vi "Asylum_Driver_LithographyObjectPoints.vi"(6 "Interpolation":dbl format="%#_13g", 7 "Writing Setpoint":dbl=0.1 format="%#_13g", 8 "error in (no error)":errorcluster, 9 "Offsets":cluster{"X":dbl, "Y":dbl}, 10 "Pattern Data":T2={"Name"="", "Litho"=[], "Set Resistance"=enum."1G ohm"}, 11 "Application":refnum<k7>) -> (0 "error out":errorcluster, 3 "Application":refnum<k7>)   [LabVIEW 2020]
uses:
  Asylum_Driver_XYMetersToVoltageArray.vi
  <userlib>/LevyLab/Relay Box/Type_defs/Resistor--enum.ctl
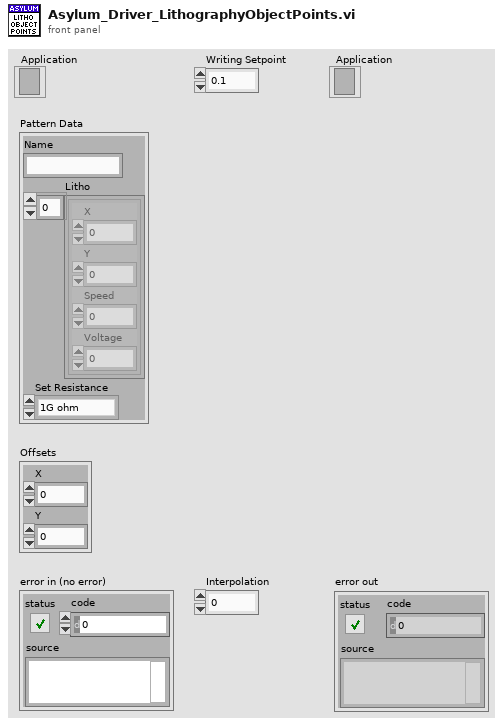
[diagram p1: front panel]
types:
  T1 = typedef "Resistor--enum.ctl" = enum16{"open", "discharge tip", "0 ohms", "100k ohm", "10M ohm", "1G ohm"}
  T2 = cluster{"Name":string, "Litho":cluster{"X":dbl, "Y":dbl, "Speed":dbl, "Voltage":dbl}[], "Set Resistance":T1}
  T3 = cluster{"setpoint":dbl, "pgain":dbl, "igain":dbl, "sgain":dbl}
  T4 = cluster{"X":dbl, "Y":dbl, "Speed":dbl, "Voltage":dbl}[]
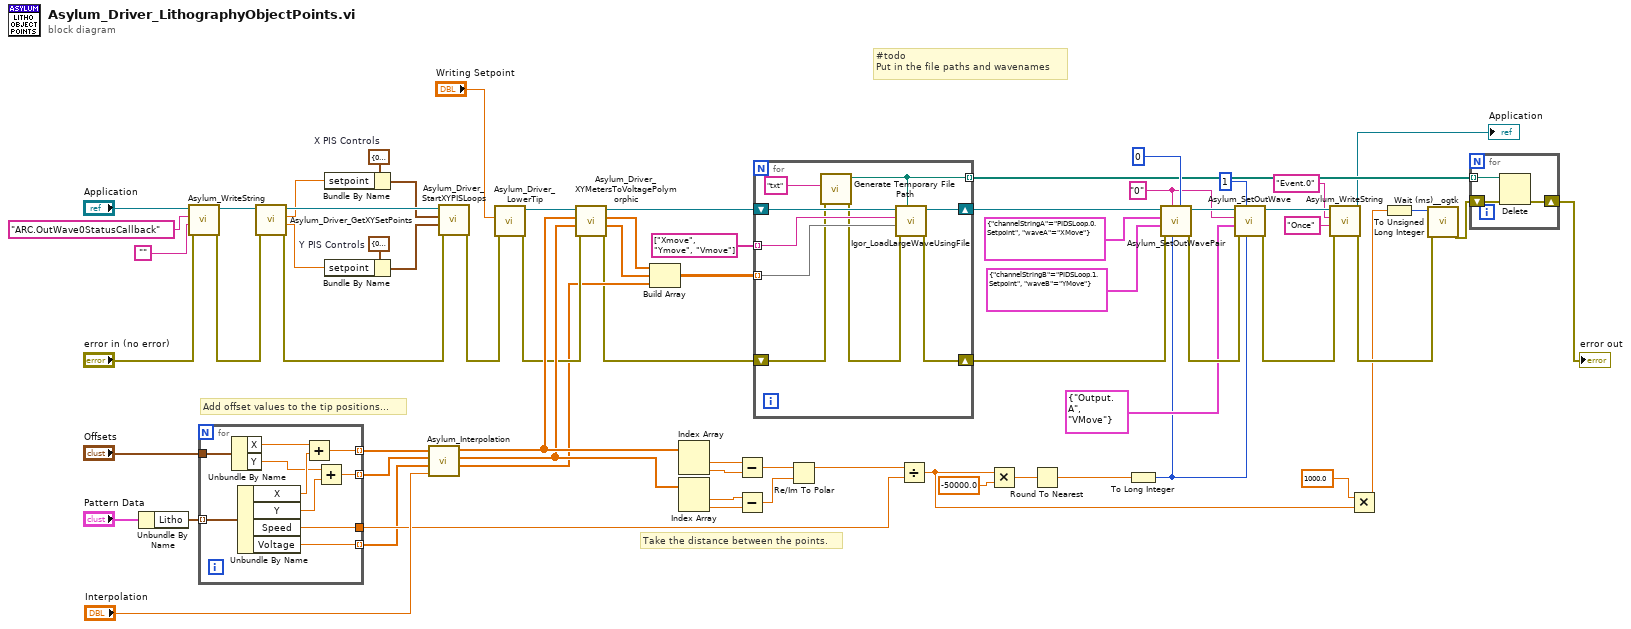
[diagram p0: block diagram]
diagram:
  w7 = "0" ("eventString")
  w63 = T3 {"setpoint"=0.0, "pgain"=0.0, "igain"=0.0, "sgain"=0.0}  # Y PIS Controls
  w64 = T3 {"setpoint"=0.0, "pgain"=0.0, "igain"=0.0, "sgain"=0.0}  # X PIS Controls
  # "Add offset values to the tip positions..."
  # "Take the distance between the points."
  # "#todo\nPut in the file paths and wavenames"
  n1 = Unbundle By Name("Pattern Data") -> ("Litho"=w68:T4)
  n2 = call <vilib>:"Asylum_WriteString.vi"("error in (no error)"="error in (no error)", "valueString"="", "parameterName"="ARC.OutWave0StatusCallback", "Application"="Application") -> ("error out"=w57:errorcluster, "Application"=w58:refnum<k7>)  [unwired: 6 in]
  n3 = for {
    tunnel: w68 -> [w79] mode=indexing
    tunnel: [w78] -> w34
    tunnel: [w77] -> w14 mode=indexing
    tunnel: "Offsets" -> [w75]
    tunnel: [w71] -> w51 mode=indexing
    tunnel: [w70] -> w45 mode=indexing
    n4 = Unbundle By Name(w75) -> ("X"=w73:dbl, "Y"=w72:dbl)
    n5 = Unbundle By Name(w79) -> ("X"=w76:dbl, "Y"=w74:dbl, "Speed"=w78:dbl, "Voltage"=w77:dbl)
    n6 = Add(x=w73, y=w76) -> (x+y=w71:dbl)
    n7 = Add(x=w72, y=w74) -> (x+y=w70:dbl)
  }
  n8 = call "Asylum_Driver_GetXYSetPoints.vi"("error in (no error)"=w57, "Application"=w58) -> ("error out"=w59:errorcluster, "Y Setpoint"=w62:dbl, "X Setpoint"=w65:dbl, "Application"=w66:refnum<k7>)  [unwired: 6 in]
  n9 = Bundle By Name(cluster=w64, "setpoint"=w65) -> (w60:T3)
  n10 = Bundle By Name(cluster=w63, "setpoint"=w62) -> (w61:T3)
  n11 = call "Asylum_Interpolation.vi"("X"=w51, "Y"=w45, "V"=w14, "Interpolation"="Interpolation") -> ("X"=w43:dbl[], "Y"=w42:dbl[], "V"=w13:dbl[])  [unwired: 4 in]
  n12 = call "Asylum_Driver_StartXYPISLoops.vi"("error in (no error)"=w59, "Y PIS Controls"=w61, "X PIS Controls"=w60, "Application"=w66) -> ("error out"=w3:errorcluster)  [unwired: 6 in, 1 out]
  n13 = call "Asylum_Driver_LowerTip.vi"("error in (no error)"=w3, "Z Setpoint"="Writing Setpoint") -> ("error out"=w27:errorcluster, "Application"=w49:refnum<k7>)  [unwired: 8 in]
  n14 = call-poly "Asylum_Driver_XYMetersToVoltagePolymorphic.vi"("error in (no error)"=w27, "Y Coordinate"=w42, "X Coordinate"=w43, "Application"=w49) -> ("error out"=w12:errorcluster, "Y Voltage"=w46:dbl[], "X Voltage"=w47:dbl[], "Application"=w48:refnum<k7>)  [unwired: 4 in]
  n15 = Build Array(w47, w46, w13) -> (w52:dbl[][])
  n16 = Index Array(array=w43) -> (element #1=w41:dbl, element #2=w40:dbl)  [unwired: 2 in]
  n17 = Index Array(array=w42) -> (element #1=w39:dbl, element #2=w38:dbl)  [unwired: 2 in]
  n18 = Subtract(x=w41, y=w40) -> (x-y=w37:dbl)
  n19 = Subtract(x=w39, y=w38) -> (x-y=w36:dbl)
  n20 = for {
    tunnel: w52 -> [w87] mode=indexing
    shift-right: [w84] -> w31
    shift-left: w12 -> [w82]
    tunnel: string[] ["Xmove", "Ymove", "Vmove"] -> [w86] mode=indexing
    shift-right: [w85] -> w29
    shift-left: w48 -> [w88]
    tunnel: [w80] -> w6 mode=indexing
    n21 = call <vilib>:"Generate Temporary File Path.vi"("error in (no error)"=w82, "Temporary File Extension (tmp)"="txt") -> ("error out"=w81:errorcluster, "Unique Temporary File Path"=w80:path)  [unwired: 8 in]
    n22 = call "Igor_LoadLargeWaveUsingFile.vi"("Path"=w80, "error in"=w81, "Wave"=w87, "Wavename"=w86, "Application"=w88) -> ("error out"=w84:errorcluster, "Application"=w85:refnum<k7>)  [unwired: 5 in]
  }
  n23 = Re/Im To Polar(2:w36, 3:w37) -> (1:w35:dbl)  [unwired: 1 out]
  n24 = Divide(x=w35, y=w34) -> (x/y=w16:dbl)
  n25 = Multiply(x=w16, y=-50000.0) -> (x*y=w32:dbl)
  n26 = Round To Nearest(number=w32) -> (nearest integer value=w11:dbl)
  n27 = To Long Integer(number=w11) -> (32bit integer=w10:i32)
  n28 = call <vilib>:"Asylum_SetOutWavePair.vi"("whichBank"=0, "interpolation"=w10, "eventString"=w7, "error in (no error)"=w31, "Wave B"=cluster{"channelStringB":string, "waveB":string} {"channelStringB"="PIDSLoop.1.Setpoint", "waveB"="YMove"}, "Wave A"=cluster{"channelStringA":string, "waveA":string} {"channelStringA"="PIDSLoop.0.Setpoint", "waveA"="XMove"}, "Application"=w29) -> ("error out"=w25:errorcluster, "Application"=w23:refnum<k7>)  [unwired: 3 in]
  n29 = call <vilib>:"Asylum_SetOutWave.vi"("interpolation"=w10, "whichBank"=1, "error in (no error)"=w25, "Wave"=cluster{"channelString":string, "wave":string} {"channelString"="Output.A", "wave"="VMove"}, "eventString"=w7, "Application"=w23) -> ("error out"=w21:errorcluster, "Application"=w20:refnum<k7>)  [unwired: 4 in]
  n30 = call <vilib>:"Asylum_WriteString.vi"("error in (no error)"=w21, "valueString"="Once", "parameterName"="Event.0", "Application"=w20) -> ("error out"=w17:errorcluster, "Application"=→"Application":refnum<k7>)  [unwired: 6 in]
  n31 = Multiply(x=1000.0, y=w16) -> (x*y=w9:dbl)
  n32 = To Unsigned Long Integer(number=w9) -> (unsigned 32bit integer=w8:u32)
  n33 = call <userlib>:"Wait (ms)__ogtk.vi"("error in (no error)"=w17, "milliseconds to wait"=w8) -> ("error out"=w5:errorcluster)  [unwired: 8 in, 1 out]
  n34 = for {
    tunnel: w6 -> [w91] mode=indexing
    shift-right: [w89] -> w4
    shift-left: w5 -> [w90]
    n35 = Delete(path (use dialog)=w91, error in=w90) -> (error out=w89:errorcluster)  [unwired: 3 in, 2 out]
  }
  "error out" <- w4
